vi "txt in current_folder.vi"(7 "file name":string) -> (8 "Path":path)   [LabVIEW 2012]
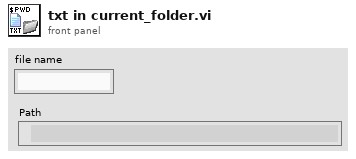
[diagram p1: front panel]
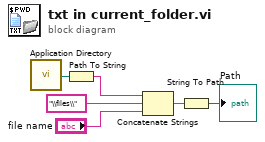
[diagram p0: block diagram]
diagram:
  n1 = call <vilib>:"Application Directory.vi"() -> ("Application Directory"=w3:path)
  n2 = Path To String(path=w3) -> (string=w1:string)
  n3 = Concatenate Strings(w1, "\\files\\" ("string"), "file name") -> (w4:string)
  n4 = String To Path(string=w4) -> (path=→"Path":path)
